vi "Multirecord Acquisition (FPGA)_20220927.vi"() -> ()   [LabVIEW 2021]
doc: "Use this VI as a template for the reconfigurable oscilloscope acquisition design. The block diagram is divided into three main loops.\n\nRegister Bus: This loop initializes the registers that are needed to support the configuration of the device. The FIFO bus, on the left, allows all the other design libraries to communicate with one another. This loop is very important to support the proper behavior of the instrument design library components.\n\nAcquisition: Acquires data from the I/O channels and writes the data into the record memory using the <B>Write</B> VI of the Multirecord Acquisition instrument design library. This VI also evaluates the various acquisition triggers and decides whether to acquire each data value in record memory. The host level VI (Fetch Record.vi) can read acquired records from the DRAM. The data is stored in 2 DRAM banks, each with 768 MB of storage.\n\nFetch: The recorded data is retrieved when the <B>Fetch Single Record</B> VI is run from the host VI. The <B>Write to Fetch DMA FIFO</B> VI writes data to the acq.fetch fifo 0 to transmit record data form the FPGA to the record fetch VIs on the host. This DMA FIFO must have a predefined name based on the instance parameter. By default, it is 0 (since the associated terminal on the <B>Create Resources DRAM Write Read</B> VI is unwired), so the connected FIFO is named acq.fetch fifo 0."
uses:
  <vilib>/Platform/TimedLoop/XDataNode/XDataNode.xnode
  <vilib>/Platform/TimedLoop/XDataNode/nitl_modes.ctl
  <vilib>/Platform/TimedLoop/XDataNode/XDNodeRunTimeDep.lvlib
  <vilib>/Platform/TimedLoop/XDataNode/wakeup.ctl
  <vilib>/Platform/TimedLoop/XDataNode/timing_clust.ctl
  <instrlib>/_niInstr/Multirecord Acquisition/Interface/v1/FPGA/niInstr Multirecord Acquisition v1 FPGA.lvclass
  <instrlib>/_niInstr/Multirecord Acquisition/Common/v1/FPGA/niInstr Multirecord Acquisition Common v1 FPGA.lvclass
  <vilib>/rvi/LocalResourceManager/LocalResourceManager.xnode
  <vilib>/rvi/eio/common/nirviEmuReportErrorAndStop.vi
  <vilib>/rvi/DataTransferAndStorage/Container/Common/niFpgaContainerGetUniqueNameForEmu.vi
  <vilib>/rvi/DataTransferAndStorage/Container/Common/niFpgaContainerSetEmuInfo.vi
  <vilib>/eio/EIONode/EIONode.xnode
  <instrlib>/_niInstr/FIFO Register Bus/v1/FPGA/niInstr FIFO Register Bus v1 FPGA.lvclass
  <instrlib>/_niInstr/Instruction Framework/v1/FPGA/Top Level Bus/Register Configuration/Register Configuration.lvclass
  <instrlib>/_niInstr/Channel/v1/FPGA/niInstr Channel v1 FPGA.lvlib
  <instrlib>/_niInstr/Basic Elements/v1/FPGA/niInstr Basic Elements v1 FPGA.lvlib
  <instrlib>/_niInstr/Multirecord Acquisition/Common/v1/FPGA/Private/Create Fetch DMA FIFO Resources U8x32.vi
  <instrlib>/HSAI-RIO/Config/Group A/v1/FPGA/Digital Correction/Digital Correction.lvclass
  <instrlib>/HSAI-RIO/Config/Group A/v1/FPGA/Config Registers/Config Registers.lvclass
  <instrlib>/_niInstr/Channel/v1/FPGA/Private/Select/Select FXP(+-,18,1,)xNspcx8ch.vi
  Trigger/Trigger FXP(+,-,18,1).vi
  Data Type Conversion/SubVIs/Remove Overflow FXP(+-,18,1)x8ch.vi
  <instrlib>/HSAI-RIO/Config/Group A/v1/FPGA/Digital Correction/FIR Filter (8 Ch).vi
  <instrlib>/_niInstr/Multirecord Acquisition/Interface/v1/FPGA/Private/Retrieve Record U16 Wrapper.vi
  <instrlib>/_niInstr/Multirecord Acquisition/Common/v1/FPGA/Private/Create Resources BRAM U384.vi
  <instrlib>/_niInstr/Multirecord Acquisition/Interface/v1/FPGA/Private/Write to Fetch DMA FIFO U16 Wrapper.vi
  <instrlib>/_niInstr/Multirecord Acquisition/Common/v1/FPGA/Private/Create Resources DRAM U384x2 U768 Write Read.vi
  Emulation/SubVIs/2 Element Generate Sine Cos Data FXP(+,-,14,1).vi
  <instrlib>/HSAI-RIO/Config/Group A/v1/FPGA/Digital Correction/Validate 8 Channel Data.vi
  <instrlib>/HSAI-RIO/Config/Group A/v1/FPGA/Digital Correction/Digital Correction (8 Ch).vi
  <instrlib>/_niInstr/Multirecord Acquisition/Common/v1/FPGA/Private/Create Resources DRAM U384.vi
  Data Type Conversion/SubVIs/Data Type Conversion FXP(+-,18,1) to I16x8ch.vi
  <instrlib>/_niInstr/Multirecord Acquisition/Common/v1/FPGA/Private/Create Resources BRAM U768.vi
  DSP/SubVIs/Integer decimationx8ch.vi
  <instrlib>/_niInstr/Multirecord Acquisition/Interface/v1/FPGA/Private/Write I16 Wrapper.vi
  <instrlib>/_niInstr/Channel/v1/FPGA/Private/Select and Interleave/Select And Interleave I16xNspcx8ch.vi
  C:/Program Files (x86)/National Instruments/LabVIEW 2021/instr.lib/_niInstr/Multirecord Acquisition/Interface/v1/FPGA/niInstr Multirecord Acquisition v1 FPGA.lvclass
  C:/Program Files (x86)/National Instruments/LabVIEW 2021/instr.lib/_niInstr/Multirecord Acquisition/Common/v1/FPGA/niInstr Multirecord Acquisition Common v1 FPGA.lvclass
  <vilib>/rvi/eio/common/nirviEmuTemplateMethod_errors.vi
  C:/Program Files (x86)/National Instruments/LabVIEW 2021/instr.lib/_niInstr/Instruction Framework/v1/FPGA/Interfaces/Instruction Producer/Instruction Producer.lvclass
  C:/Program Files (x86)/National Instruments/LabVIEW 2021/instr.lib/_niInstr/FIFO Register Bus/v1/FPGA/niInstr FIFO Register Bus v1 FPGA.lvclass
  FPGA Interface Typedefinitions/Trigger Combination Type.ctl
  FPGA Interface Typedefinitions/FPGA Interface Typedefinitions.lvlib
  <instrlib>/_niInstr/Data Trigger/v1/Shared/Public/Level Configuration FXP(+-,18,1).ctl
  <instrlib>/_niInstr/Data Trigger/v1/Shared/niInstr Data Trigger v1 Shared.lvlib
  <instrlib>/_niInstr/Data Trigger/v1/Shared/Public/Level Configuration Trigger When.ctl
panel:
  in  "trig 0":cluster{"Hi":T1, "Lo":T1}
  in  "trigger.channel A":u8
  in  "trigger.rearm delay":u16=2
  in  "start trigger":bool=TRUE
  in  "reset":bool
  in  "trigger.combination type":T3
  out "fifo reg bus data 0":u64
  out "fifo reg bus status 0":u32
  in  "fifo reg bus ctrl 0":u32
  out "overflow":bool
  in  "dsp.decimation factor":u16
  out "overload":bool
  in  "channel.enable mask":u16=65535 format="%.0b"
  in  "channel.number of channels":u8=8
  # "Register Bus Controls"
  # "FPGA"
  # "Acquisition Loop Controls"
  # "DSP"
  # "Trigger"
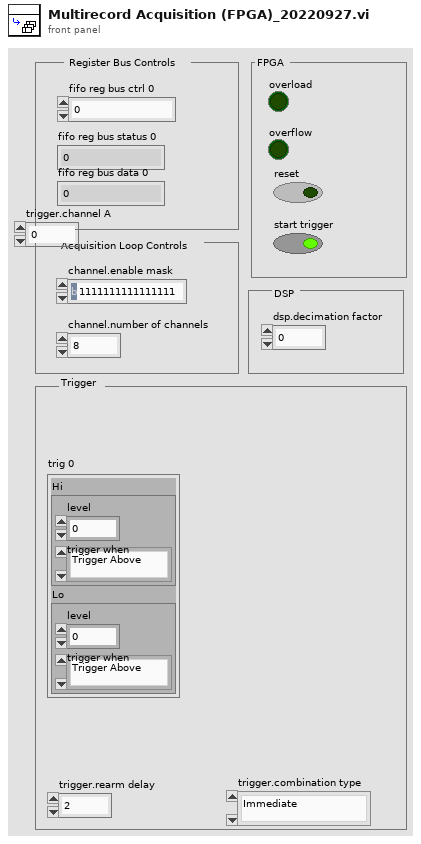
[diagram p1: front panel]
types:
  T1 = typedef "niInstr Data Trigger v1 Shared.lvlib/Level Configuration FXP(+-,18,1).ctl" = cluster{"level":fxp<+/-,18,1>, "trigger when":T2}
  T2 = typedef "niInstr Data Trigger v1 Shared.lvlib/Level Configuration Trigger When.ctl" = enum8{"Trigger Above", "Trigger Below"}
  T3 = typedef "FPGA Interface Typedefinitions.lvlib/Trigger Combination Type.ctl" = enum16{"Immediate", "A", "B", "OR", "AND", "A THEN B", "B THEN A", "High Resolution"}
  T4 = cluster{"memory 1":refnum<k21>, "memory 2":refnum<k21>}
  T5 = typedef "XDNodeRunTimeDep.lvlib/timing_clust.ctl" = cluster{"Expected End [f-1]":u64, "Actual End [f-1]":u64, "Finished Late? [f-1]":bool, "Expected End [i-1]":u64, "Actual End [i-1]":u64, "Finished Late? [i-1]":bool, "Expected Start [i]":u64, "Actual Start [i]":u64, "Expected Start [f]":u64, "Actual Start [f]":u64, "Source Name":string, "Structure Name":string, "Period":i64, "Deadline":i64, "Offset":i64, "Start":i64, "Priority":i32, "Timeout":i32, "Mode":T6, "Wakeup Reason":T7, "Error":errorcluster, "Source Type":string, "Secondary Source Type":string, "Global End Time":u64, "Global Start Time":u64, "Frame Duration":u64, "Iteration Duration":u64, "Assigned CPU":i32, "I/O Scan Engine Mode":u32}
  T6 = typedef "XDNodeRunTimeDep.lvlib/nitl_modes.ctl" = enum32{"No Change", "Process missed periods, maintain original phase", "Discard missed periods, maintain original phase", "Process missed periods, ignore original phase", "Discard missed periods, ignore original phase"}
  T7 = typedef "XDNodeRunTimeDep.lvlib/wakeup.ctl" = enum32{"Normal", "Aborted", "Asynchronous wakeup", "Timing source error", "Timed loop error", "Timeout"}
  T8 = cluster{"sine data":fxp<+/-,14,1>[], "cosine data":fxp<+/-,14,1>[], "sine data":fxp<+/-,14,1>[], "cosine data":fxp<+/-,14,1>[], "sine data":fxp<+/-,14,1>[], "cosine data":fxp<+/-,14,1>[], "sine data":fxp<+/-,14,1>[], "cosine data":fxp<+/-,14,1>[]}
  T9 = cluster{"Channel 0":fxp<+/-,18,1>[], "Channel 1":fxp<+/-,18,1>[], "Channel 2":fxp<+/-,18,1>[], "Channel 3":fxp<+/-,18,1>[], "Channel 4":fxp<+/-,18,1>[], "Channel 5":fxp<+/-,18,1>[], "Channel 6":fxp<+/-,18,1>[], "Channel 7":fxp<+/-,18,1>[]}
  T10 = cluster{"channel 0":fxp<+/-,18,1>[], "channel 1":fxp<+/-,18,1>[], "channel 2":fxp<+/-,18,1>[], "channel 3":fxp<+/-,18,1>[], "channel 4":fxp<+/-,18,1>[], "channel 5":fxp<+/-,18,1>[], "channel 6":fxp<+/-,18,1>[], "channel 7":fxp<+/-,18,1>[]}
  T11 = cluster{"channel 0":i16[], "channel 1":i16[], "channel 2":i16[], "channel 3":i16[], "channel 4":i16[], "channel 5":i16[], "channel 6":i16[], "channel 7":i16[]}
  T12 = typedef "niInstr Multirecord Acquisition v1 FPGA.lvclass/Timestamp.ctl" = cluster{"timestamp":u64, "valid":bool}
  T13 = typedef "niInstr Types v1 Shared.lvlib/Input Triggers.ctl" = cluster{"start":bool, "advance":bool, "reference":bool, "start trigger index":u16, "advance trigger index":u16, "reference trigger index":u16, "reference trigger correction cycle count":u32}
  T14 = typedef "niInstr Types v1 Shared.lvlib/Sample Format.ctl" = cluster{"bits per channel":u16, "samples per clock":u16, "channels":u8}
  T15 = typedef "niInstr Multirecord Acquisition v1 FPGA.lvclass/Events.ctl" = cluster{"ready for start":bool, "ready for advance":bool, "ready for reference":bool, "end of record":bool, "done":bool, "start trigger":bool, "advance trigger":bool, "reference trigger":bool, "start trigger index":u16, "advance trigger index":u16, "reference trigger index":u16}
  T16 = typedef "niInstr Multirecord Acquisition v1 FPGA.lvclass/Retrieve Data Info.ctl" = cluster{"read request size (bits)":u64, "valid data offset (bits)":u16, "valid data size (bits)":u16, "first sample of request":bool, "last sample of request":bool, "Token":T17}
  T17 = typedef "niInstr Types v1 Shared.lvlib/Token.ctl" = cluster{"identifier":u8, "value":u32}
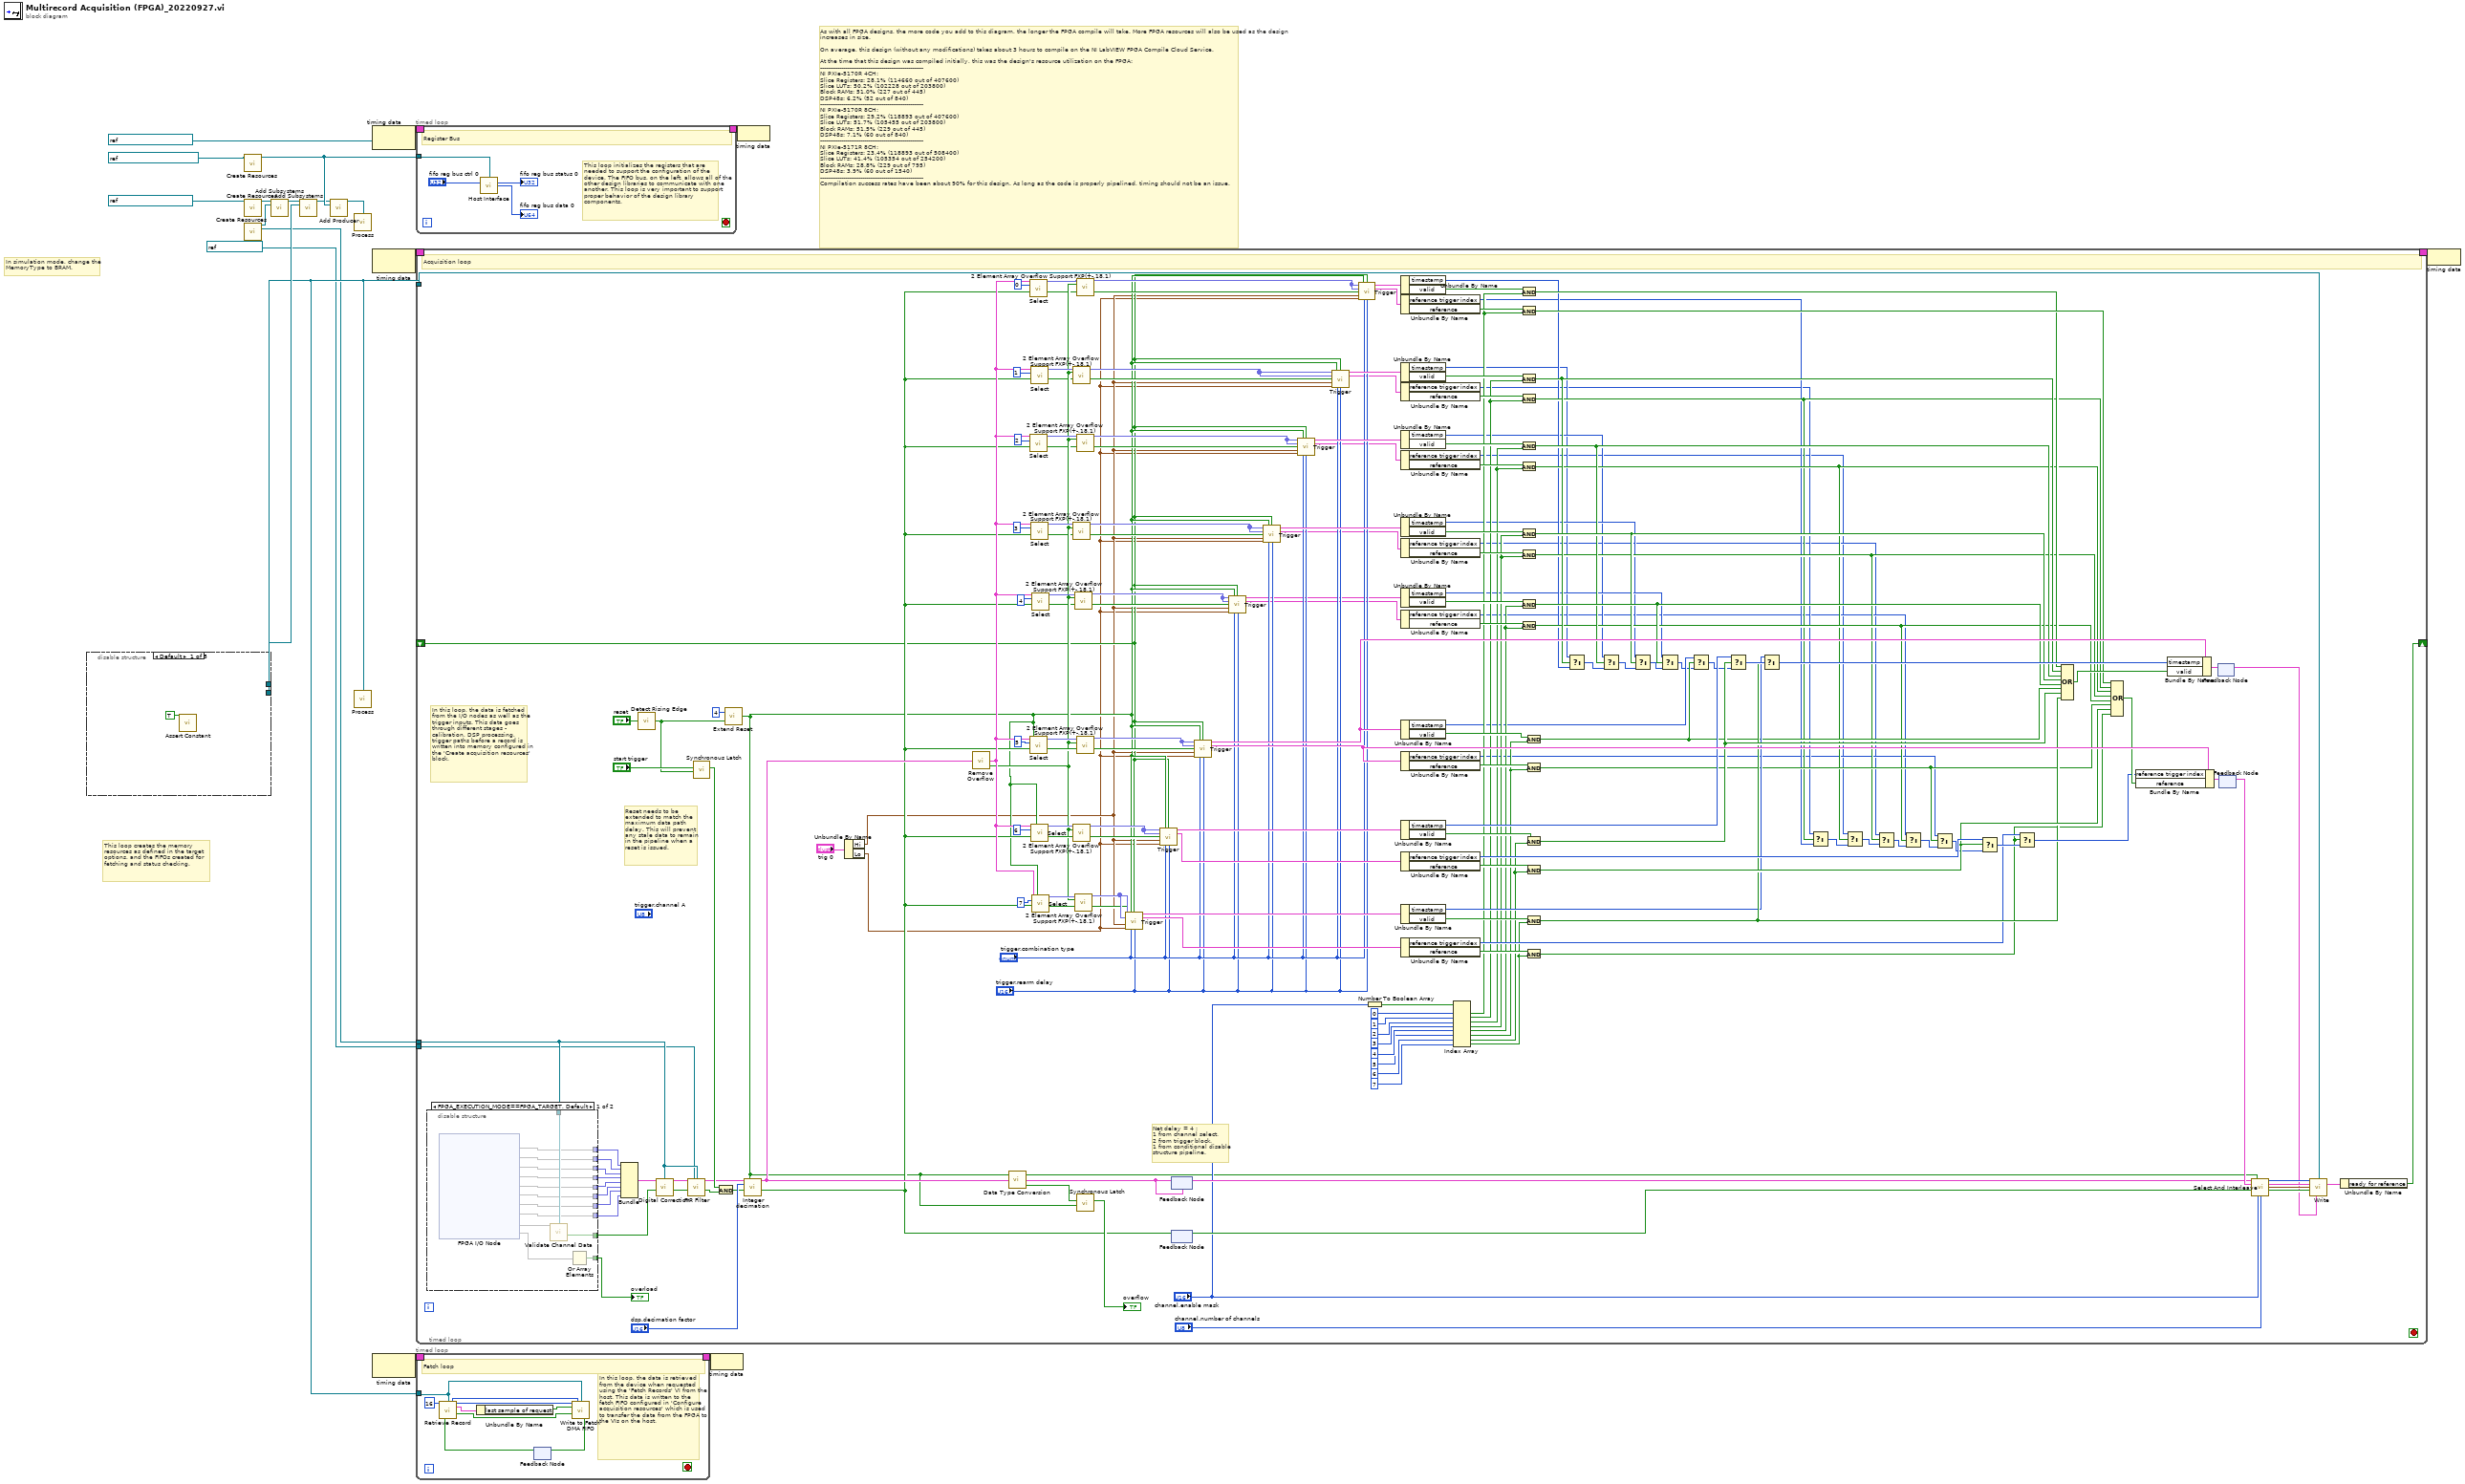
[diagram p0: block diagram]
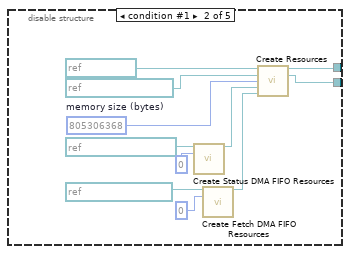
[diagram p2: hidden frame]
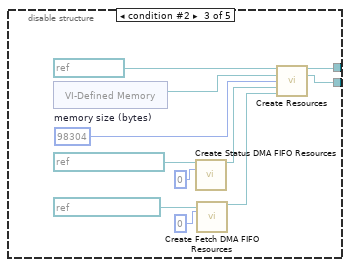
[diagram p3: hidden frame]
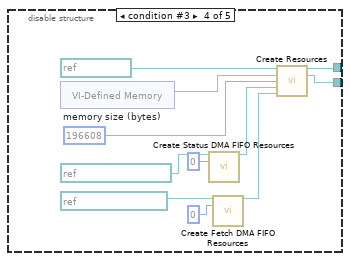
[diagram p4: hidden frame]
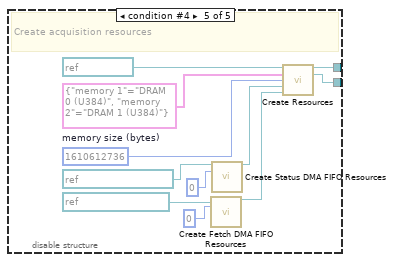
[diagram p5: hidden frame]
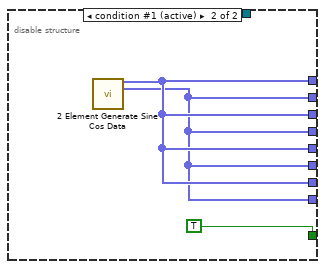
[diagram p6: hidden frame]
diagram:
  # "In simulation mode, change the MemoryType to BRAM."
  # "This loop creates the memory resources as defined in the target options, and the FIFOs created for fetching and status checking."
  # "As with all FPGA designs, the more code you add to this diagram, the longer the FPGA compile will take. More FPGA resources will also be used as the design increases in size.\n\nOn average, this design (without any modifications) takes about 3 hours to compile on the NI LabVIEW FPGA Compile Cloud Service. \n\nAt the time that this design was compiled initially, this was the design's resource utilization on the FPGA:\n------------------------------------------------------\nNI PXIe-5170R 4CH:\nSlice Registers: 28.1% (114660 out of 407600)\nSlice LUTs: 50.2% (102228 out of 203800)\nBlock RAMs: 51.0% (227 out of 445)\nDSP48s: 6.2% (52 out of 840)\n------------------------------------------------------\nNI PXIe-5170R 8CH:\nSlice Registers: 29.2% (118893 out of 407600)\nSlice LUTs: 51.7% (105455 out of 203800)\nBlock RAMs: 51.5% (229 out of 445)\nDSP48s: 7.1% (60 out of 840)\n------------------------------------------------------\nNI PXIe-5171R 8CH:\nSlice Registers: 23.4% (118893 out of 508400)\nSlice LUTs: 41.4% (105354 out of 254200)\nBlock RAMs: 28.8% (229 out of 795)\nDSP48s: 3.9% (60 out of 1540)\n------------------------------------------------------\nCompilation success rates have been about 90% for this design. As long as the code is properly pipelined, timing should not be an issue."
  n1 = disable-structure shown="Default" {
    disable-tunnel: [_ w29 w40 w51 w62] -> w4
    disable-tunnel: [_ w26 w36 w47 w59] -> w7
    frame condition #0 (active) {
      n2 = call <instrlib>:"Assert Constant.vi"("constant terminal"=TRUE) -> ()  [unwired: 15 in]
    }
    frame condition #1 {
      w30 = u64 805306368  # memory size (bytes)
      n3 = call <instrlib>:"Create Status DMA FIFO Resources.vi"("status dma fifo in"=refnum<k21> "acq.status fifo 0" ("status dma fifo"), "fifo instance"=u8 0) -> ("status dma fifo out"=w21:refnum<class "niInstr Status FIFO v1 FPGA.lvclass">)  [unwired: 13 in]
      n4 = call-poly <instrlib>:"Create Fetch DMA FIFO Resources.vi"("fetch dma fifo in"=refnum<k21> "acq.fetch fifo 0", "fifo instance"=u8 0) -> ("fetch dma fifo out"=w27:refnum<class "niInstr Fetch FIFO v1 FPGA.lvclass">)  [unwired: 13 in]
      n5 = call-poly <instrlib>:"Create Resources.vi"("memory clock"=refnum<k21> "160MHz" ("process clock"), "memory"=refnum<k21> "DRAM 0 (U384)" ("dram"), "memory size (bytes)"=w30, "status dma fifo resources"=w21, "fetch dma fifo resources"=w27) -> ("acquisition resources"=w29:refnum<class "niInstr Multirecord Acquisition Common v1 FPGA.lvclass">, "acquisition subsystem"=w26:refnum<class "Address Space Collection.lvclass">)  [unwired: 9 in]
    }
    frame condition #2 {
      w41 = u64 98304  # memory size (bytes)
      n6 = xnode "VI-Defined Memory"() -> ("Memory Out"=w42:refnum<k21>)
      n7 = call <instrlib>:"Create Status DMA FIFO Resources.vi"("status dma fifo in"=refnum<k21> "acq.status fifo 0" ("status dma fifo"), "fifo instance"=u8 0) -> ("status dma fifo out"=w33:refnum<class "niInstr Status FIFO v1 FPGA.lvclass">)  [unwired: 13 in]
      n8 = call-poly <instrlib>:"Create Fetch DMA FIFO Resources.vi"("fetch dma fifo in"=refnum<k21> "acq.fetch fifo 0", "fifo instance"=u8 0) -> ("fetch dma fifo out"=w37:refnum<class "niInstr Fetch FIFO v1 FPGA.lvclass">)  [unwired: 13 in]
      n9 = call-poly <instrlib>:"Create Resources.vi"("memory clock"=refnum<k21> "160MHz" ("process clock"), "memory"=w42, "memory size (bytes)"=w41, "status dma fifo resources"=w33, "fetch dma fifo resources"=w37) -> ("acquisition resources"=w40:refnum<class "niInstr Multirecord Acquisition Common v1 FPGA.lvclass">, "acquisition subsystem"=w36:refnum<class "Address Space Collection.lvclass">)  [unwired: 9 in]
    }
    frame condition #3 {
      w52 = u64 196608  # memory size (bytes)
      n10 = xnode "VI-Defined Memory"() -> ("Memory Out"=w53:refnum<k21>)
      n11 = call <instrlib>:"Create Status DMA FIFO Resources.vi"("status dma fifo in"=refnum<k21> "acq.status fifo 0" ("status dma fifo"), "fifo instance"=u8 0) -> ("status dma fifo out"=w45:refnum<class "niInstr Status FIFO v1 FPGA.lvclass">)  [unwired: 13 in]
      n12 = call-poly <instrlib>:"Create Fetch DMA FIFO Resources.vi"("fetch dma fifo in"=refnum<k21> "acq.fetch fifo 0", "fifo instance"=u8 0) -> ("fetch dma fifo out"=w48:refnum<class "niInstr Fetch FIFO v1 FPGA.lvclass">)  [unwired: 13 in]
      n13 = call-poly <instrlib>:"Create Resources.vi"("memory clock"=refnum<k21> "160MHz" ("process clock"), "memory"=w53, "memory size (bytes)"=w52, "status dma fifo resources"=w45, "fetch dma fifo resources"=w48) -> ("acquisition resources"=w51:refnum<class "niInstr Multirecord Acquisition Common v1 FPGA.lvclass">, "acquisition subsystem"=w47:refnum<class "Address Space Collection.lvclass">)  [unwired: 9 in]
    }
    frame condition #4 {
      w64 = u64 1610612736  # memory size (bytes)
      # "Create acquisition resources"
      n14 = call-poly <instrlib>:"Create Fetch DMA FIFO Resources.vi"("fetch dma fifo in"=refnum<k21> "acq.fetch fifo 0", "fifo instance"=u8 0) -> ("fetch dma fifo out"=w61:refnum<class "niInstr Fetch FIFO v1 FPGA.lvclass">)  [unwired: 13 in]
      n15 = call <instrlib>:"Create Status DMA FIFO Resources.vi"("status dma fifo in"=refnum<k21> "acq.status fifo 0" ("status dma fifo"), "fifo instance"=u8 0) -> ("status dma fifo out"=w56:refnum<class "niInstr Status FIFO v1 FPGA.lvclass">)  [unwired: 13 in]
      n16 = call-poly <instrlib>:"Create Resources.vi"("memory clock"=refnum<k21> "160MHz" ("process clock"), "memory"=T4 {"memory 1"="DRAM 0 (U384)", "memory 2"="DRAM 1 (U384)"}, "memory size (bytes)"=w64, "status dma fifo resources"=w56, "fetch dma fifo resources"=w61) -> ("acquisition resources"=w62:refnum<class "niInstr Multirecord Acquisition Common v1 FPGA.lvclass">, "acquisition subsystem"=w59:refnum<class "Address Space Collection.lvclass">)  [unwired: 9 in]
    }
  }
  n17 = call <instrlib>:"Create Resources.vi"("instruction fifo"=refnum<k21> "reg.host instruction fifo 0" ("FIFO")) -> ("fifo register bus"=w6:refnum<class "niInstr FIFO Register Bus v1 FPGA.lvclass">)  [unwired: 14 in]
  n18 = call <instrlib>:"Create Resources.vi"("register clock"=refnum<k21> "40 MHz Onboard Clock" ("Source Name")) -> ("register configuration"=w10:refnum<class "Register Configuration.lvclass">)  [unwired: 14 in]
  n19 = call <instrlib>:"Create Resources.vi"() -> ("config subsystems"=w8:refnum<class "Address Space Collection.lvclass">, "digital correction resources"=w1:refnum<class "Digital Correction.lvclass">)  [unwired: 14 in]
  n20 = call-dynamic "Add Subsystems.vi"("register configuration in"=w10, "subsystems"=w8) -> ("register configuration out"=w9:refnum<class "Register Configuration.lvclass">)  [unwired: 13 in]
  n21 = call-dynamic "Add Subsystems.vi"("register configuration in"=w9, "subsystems"=w7) -> ("register configuration out"=w3:refnum<class "Register Configuration.lvclass">)  [unwired: 13 in]
  n22 = call-dynamic "Add Producer.vi"("register configuration in"=w3, "instruction producer"=w6) -> ("register configuration out"=w5:refnum<class "Register Configuration.lvclass">)  [unwired: 13 in]
  n23 = call-dynamic "Process.vi"("register configuration"=w5) -> ()  [unwired: 15 in]
  n24 = call-dynamic "Process.vi"("acquisition resources"=w4) -> ()  [unwired: 15 in]
  n25 = node-c288(refnum<k21> "40 MHz Onboard Clock" ("Source Name")) -> (w19:T5)
  n26 = node-c288() -> (w17:T5)  [unwired: 1 in]
  n27 = node-c288() -> (w15:T5)  [unwired: 1 in]
  n28 = timed-loop {
    timing: w19 -> [_]
    timing-out: [_] -> w18
    tunnel: w6 -> [w68]
    stop <- _ stop-if-true
    # "This loop initializes the registers that are needed to support the configuration of the device. The FIFO bus, on the left, allows all of the other design libraries to communicate with one another. This loop is very important to support proper behavior of the design library components."
    # "Register Bus"
    n29 = call <instrlib>:"Host Interface.vi"("fifo register bus"=w68, "fifo reg bus ctrl 0"="fifo reg bus ctrl 0") -> ("fifo reg bus status 0"=→"fifo reg bus status 0":u32, "fifo reg bus data 0"=→"fifo reg bus data 0":u64)  [unwired: 12 in]
  }
  n30 = timed-loop {
    timing: w17 -> [_]
    timing-out: [_] -> w16
    tunnel: w4 -> [w251]
    tunnel: w1 -> [w234]
    shift-right: [w243] -> _
    shift-left: _ -> [w145]
    tunnel: refnum<k21> "Data Clock x2" -> [w231]
    stop <- _ stop-if-true
    # "Net delay = 4 :\n1 from channel select.\n2 from trigger block.\n1 from conditional disable structure pipeline."
    # "Reset needs to be extended to match the maximum data path delay. This will prevent any stale data to remain in the pipeline when a reset is issued."
    # "In this loop, the data is fetched from the I/O nodes as well as the trigger inputs. This data goes through different stages - calibration, DSP processing, trigger paths before a record is written into memory configured in the 'Create acquisition resources' block."
    # "Acquisition loop"
    n31 = disable-structure shown="FPGA_EXECUTION_MODE==FPGA_TARGET, Default" {
      disable-tunnel: [w263 w268] -> w230
      disable-tunnel: [w262 w267] -> w229
      disable-tunnel: [w261 w268] -> w228
      disable-tunnel: [w260 w267] -> w227
      disable-tunnel: [w259 w268] -> w226
      disable-tunnel: [w258 w267] -> w225
      disable-tunnel: [w257 w268] -> w223
      disable-tunnel: [w256 w267] -> w224
      disable-tunnel: [w253 TRUE ("ADC Data Valid")] -> w221
      disable-tunnel: w234 -> [w264 _]
      disable-tunnel: [w254 _] -> w250
      frame condition #0 {
        # "I/O Nodes"
        n32 = xnode "FPGA I/O Node"() -> ("Channel 0"=w263, "Channel 1"=w262, "Channel 2"=w261, "Channel 3"=w260, "Channel 4"=w259, "Channel 5"=w258, "Channel 6"=w257, "Channel 7"=w256, "Channel Data Valid"=w265, "Channel Overload"=w255)  [unwired: 10 in, 10 out]
        n33 = call-poly <instrlib>:"Validate Channel Data.vi"("channel data valid"=w265, "digital correction resources"=w264) -> ("expected data valid"=w253:bool)  [unwired: 13 in]
        n34 = Or Array Elements(Boolean array=w255) -> (logical OR=w254:bool)
      }
      frame condition #1 (active) {
        n35 = call-poly "2 Element Generate Sine Cos Data.vi"() -> ("sine data"=w268:fxp<+/-,14,1>[], "cosine data"=w267:fxp<+/-,14,1>[])  [unwired: 14 in]
      }
    }
    "overload" <- w250
    n36 = Bundle("sine data"=w230, "cosine data"=w229, "sine data"=w228, "cosine data"=w227, "sine data"=w226, "cosine data"=w225, "sine data"=w223, "cosine data"=w224) -> (w222:T8)  [unwired: 1 in]
    n37 = call <instrlib>:"Detect Rising Edge.vi"("signal"="reset") -> ("edge detected"=w233:bool)  [unwired: 14 in]
    n38 = call-poly <instrlib>:"Digital Correction.vi"("channel data in"=w222, "digital correction resources"=w234, "input valid"=w221) -> ("corrected channel data out"=w214:T9, "output valid"=w213:bool)  [unwired: 11 in]
    n39 = call-poly <instrlib>:"FIR Filter.vi"("data in"=w214, "data clock x2"=w231, "digital correction resources"=w234, "input valid"=w213) -> ("data out"=w211:T9, "output valid"=w212:bool)  [unwired: 9 in, 1 out]
    n40 = call <instrlib>:"Synchronous Latch.vi"("clear"=w233, "set"="start trigger") -> ("out"=w239:bool)  [unwired: 9 in]
    n41 = And(x=w239, y=w212) -> (x .and. y?=w215:bool)
    n42 = call "Extend Reset.vi"("reset in"=w233, "number of cycles"=u8 4) -> ("reset out"=w146:bool)
    n43 = call-poly "Integer decimation.vi"("data in"=w211, "reset"=w146, "decimation factor"="dsp.decimation factor", "input valid"=w215) -> ("data out"=w218:T10, "output valid"=w162:bool)  [unwired: 9 in, 1 out]
    n44 = Unbundle By Name("trig 0") -> ("Hi"=w72:T1, "Lo"=w71:T1)
    n45 = call-poly "Remove Overflow.vi"("data in"=w218) -> ("overflow"=w156:bool, "data out"=w168:T10)  [unwired: 3 in]
    n46 = call-poly "Data Type Conversion.vi"("data in"=w218) -> ("overflow"=w220:bool, "data out"=w217:T11)  [unwired: 3 in]
    n47 = call-poly <instrlib>:"Select.vi"("data in"=w168, "channel index"=u8 0 ("trigger.channel A"), "input valid"=w162) -> ("channel out"=w167:fxp<+/-,18,1>[], "output valid"=w151:bool)  [unwired: 11 in]
    n48 = call-poly <instrlib>:"Select.vi"("data in"=w168, "channel index"=u8 2 ("trigger.channel A"), "input valid"=w162) -> ("channel out"=w165:fxp<+/-,18,1>[], "output valid"=w153:bool)  [unwired: 11 in]
    n49 = call-poly <instrlib>:"Select.vi"("data in"=w168, "reset"=w146, "channel index"=u8 5 ("trigger.channel A"), "input valid"=w162) -> ("channel out"=w241:fxp<+/-,18,1>[], "output valid"=w210:bool)  [unwired: 10 in]
    n50 = call-poly <instrlib>:"Select.vi"("data in"=w168, "channel index"=u8 1, "input valid"=w162) -> ("channel out"=w166:fxp<+/-,18,1>[], "output valid"=w152:bool)  [unwired: 11 in]
    n51 = call-poly <instrlib>:"Select.vi"("data in"=w168, "channel index"=u8 3, "input valid"=w162) -> ("channel out"=w164:fxp<+/-,18,1>[], "output valid"=w154:bool)  [unwired: 11 in]
    n52 = call-poly <instrlib>:"Select.vi"("data in"=w168, "reset"=w146, "channel index"=u8 6, "input valid"=w162) -> ("channel out"=w207:fxp<+/-,18,1>[], "output valid"=w205:bool)  [unwired: 10 in]
    n53 = call-poly <instrlib>:"Select.vi"("data in"=w168, "channel index"=u8 4, "input valid"=w162) -> ("channel out"=w163:fxp<+/-,18,1>[], "output valid"=w155:bool)  [unwired: 11 in]
    n54 = call-poly <instrlib>:"Select.vi"("data in"=w168, "reset"=w146, "channel index"=u8 7, "input valid"=w162) -> ("channel out"=w186:fxp<+/-,18,1>[], "output valid"=w184:bool)  [unwired: 10 in]
    n55 = call "2 Element Array Overflow Support FXP(+-,18,1).vi"("data in"=w166, "overflow"=w156) -> ("data out"=w160:fxp<+/-,18,1>[])  [unwired: 13 in]
    n56 = call "2 Element Array Overflow Support FXP(+-,18,1).vi"("data in"=w164, "overflow"=w156) -> ("data out"=w158:fxp<+/-,18,1>[])  [unwired: 13 in]
    n57 = call "2 Element Array Overflow Support FXP(+-,18,1).vi"("data in"=w207, "overflow"=w156) -> ("data out"=w206:fxp<+/-,18,1>[])  [unwired: 13 in]
    n58 = call "2 Element Array Overflow Support FXP(+-,18,1).vi"("data in"=w163, "overflow"=w156) -> ("data out"=w157:fxp<+/-,18,1>[])  [unwired: 13 in]
    n59 = call "2 Element Array Overflow Support FXP(+-,18,1).vi"("data in"=w186, "overflow"=w156) -> ("data out"=w185:fxp<+/-,18,1>[])  [unwired: 13 in]
    n60 = call "2 Element Array Overflow Support FXP(+-,18,1).vi"("data in"=w167, "overflow"=w156) -> ("data out"=w161:fxp<+/-,18,1>[])  [unwired: 13 in]
    n61 = call "2 Element Array Overflow Support FXP(+-,18,1).vi"("data in"=w165, "overflow"=w156) -> ("data out"=w159:fxp<+/-,18,1>[])  [unwired: 13 in]
    n62 = call "2 Element Array Overflow Support FXP(+-,18,1).vi"("data in"=w241, "overflow"=w156) -> ("data out"=w209:fxp<+/-,18,1>[])  [unwired: 13 in]
    n63 = call <instrlib>:"Synchronous Latch.vi"("clear"=w146, "set"=w220) -> ("out"=→"overflow":bool)  [unwired: 9 in]
    n64 = call-poly "Trigger.vi"("data A"=w185, "reset"=w146, "trigger.ready for reference"=w145, "data B"=w185, "input valid"=w184, "trigger.level Hi"=w72, "trigger.level Lo"=w71, "trigger.combination type"="trigger.combination type", "rearm delay"="trigger.rearm delay") -> ("timestamps"=w183:T12, "trigger.out"=w182:T13)  [unwired: 4 in, 1 out]
    n65 = call-poly "Trigger.vi"("data A"=w206, "reset"=w146, "trigger.ready for reference"=w145, "data B"=w206, "input valid"=w205, "trigger.level Hi"=w72, "trigger.level Lo"=w71, "trigger.combination type"="trigger.combination type", "rearm delay"="trigger.rearm delay") -> ("timestamps"=w200:T12, "trigger.out"=w199:T13)  [unwired: 4 in, 1 out]
    n66 = feedback #1(w217) -> (w219:T11)
    n67 = feedback-in #1(w217) -> ()
    n68 = feedback #2() -> (w216:bool)  [unwired: 1 in]
    n69 = feedback-in #2(w162) -> ()
    n70 = call-poly "Trigger.vi"("data A"=w209, "reset"=w146, "trigger.ready for reference"=w145, "data B"=w209, "input valid"=w210, "trigger.level Hi"=w72, "trigger.level Lo"=w71, "trigger.combination type"="trigger.combination type", "rearm delay"="trigger.rearm delay") -> ("timestamps"=w204:T12, "trigger.out"=w202:T13)  [unwired: 4 in, 1 out]
    n71 = call-poly "Trigger.vi"("data A"=w157, "reset"=w146, "trigger.ready for reference"=w145, "data B"=w157, "input valid"=w155, "trigger.level Hi"=w72, "trigger.level Lo"=w71, "trigger.combination type"="trigger.combination type", "rearm delay"="trigger.rearm delay") -> ("timestamps"=w138:T12, "trigger.out"=w137:T13)  [unwired: 4 in, 1 out]
    n72 = call-poly "Trigger.vi"("data A"=w158, "reset"=w146, "trigger.ready for reference"=w145, "data B"=w158, "input valid"=w154, "trigger.level Hi"=w72, "trigger.level Lo"=w71, "trigger.combination type"="trigger.combination type", "rearm delay"="trigger.rearm delay") -> ("timestamps"=w147:T12, "trigger.out"=w139:T13)  [unwired: 4 in, 1 out]
    n73 = call-poly "Trigger.vi"("data A"=w159, "reset"=w146, "trigger.ready for reference"=w145, "data B"=w159, "input valid"=w153, "trigger.level Hi"=w72, "trigger.level Lo"=w71, "trigger.combination type"="trigger.combination type", "rearm delay"="trigger.rearm delay") -> ("timestamps"=w148:T12, "trigger.out"=w140:T13)  [unwired: 4 in, 1 out]
    n74 = call-poly "Trigger.vi"("data A"=w160, "reset"=w146, "trigger.ready for reference"=w145, "data B"=w160, "input valid"=w152, "trigger.level Hi"=w72, "trigger.level Lo"=w71, "trigger.combination type"="trigger.combination type", "rearm delay"="trigger.rearm delay") -> ("timestamps"=w149:T12, "trigger.out"=w141:T13)  [unwired: 4 in, 1 out]
    n75 = call-poly "Trigger.vi"("data A"=w161, "reset"=w146, "trigger.ready for reference"=w145, "data B"=w161, "input valid"=w151, "trigger.level Hi"=w72, "trigger.level Lo"=w71, "trigger.combination type"="trigger.combination type", "rearm delay"="trigger.rearm delay") -> ("timestamps"=w150:T12, "trigger.out"=w142:T13)  [unwired: 4 in, 1 out]
    n76 = Number To Boolean Array(number="channel.enable mask") -> (Boolean array=w195:bool[])
    n77 = Unbundle By Name(w150) -> ("timestamp"=w100:u64, "valid"=w131:bool)
    n78 = Unbundle By Name(w142) -> ("reference trigger index"=w89:u16, "reference"=w130:bool)
    n79 = Unbundle By Name(w149) -> ("timestamp"=w90:u64, "valid"=w129:bool)
    n80 = Unbundle By Name(w141) -> ("reference trigger index"=w88:u16, "reference"=w128:bool)
    n81 = Unbundle By Name(w148) -> ("timestamp"=w91:u64, "valid"=w127:bool)
    n82 = Unbundle By Name(w140) -> ("reference trigger index"=w79:u16, "reference"=w126:bool)
    n83 = Unbundle By Name(w147) -> ("timestamp"=w92:u64, "valid"=w125:bool)
    n84 = Unbundle By Name(w139) -> ("reference trigger index"=w80:u16, "reference"=w124:bool)
    n85 = Unbundle By Name(w138) -> ("timestamp"=w93:u64, "valid"=w123:bool)
    n86 = Unbundle By Name(w137) -> ("reference trigger index"=w81:u16, "reference"=w122:bool)
    n87 = Unbundle By Name(w204) -> ("timestamp"=w99:u64, "valid"=w192:bool)
    n88 = Unbundle By Name(w202) -> ("reference trigger index"=w83:u16, "reference"=w190:bool)
    n89 = Unbundle By Name(w200) -> ("timestamp"=w198:u64, "valid"=w191:bool)
    n90 = Unbundle By Name(w199) -> ("reference trigger index"=w197:u16, "reference"=w189:bool)
    n91 = Unbundle By Name(w183) -> ("timestamp"=w170:u64, "valid"=w180:bool)
    n92 = Unbundle By Name(w182) -> ("reference trigger index"=w169:u16, "reference"=w181:bool)
    n93 = Index Array(array=w195, index #1=0 ("index"), index #2=1 ("index"), index #3=2 ("index"), index #4=3 ("index"), index #5=4 ("index"), index #6=5 ("index"), index #7=6 ("index"), index #8=7 ("index")) -> (element #1=w121:bool, element #2=w120:bool, element #3=w119:bool, element #4=w118:bool, element #5=w117:bool, element #6=w116:bool, element #7=w115:bool, element #8=w114:bool)
    n94 = And(x=w131, y=w121) -> (x .and. y?=w111:bool)
    n95 = And(x=w130, y=w121) -> (x .and. y?=w112:bool)
    n96 = And(x=w129, y=w120) -> (x .and. y?=w106:bool)
    n97 = And(x=w128, y=w120) -> (x .and. y?=w101:bool)
    n98 = And(x=w127, y=w119) -> (x .and. y?=w107:bool)
    n99 = And(x=w126, y=w119) -> (x .and. y?=w102:bool)
    n100 = And(x=w125, y=w118) -> (x .and. y?=w108:bool)
    n101 = And(x=w124, y=w118) -> (x .and. y?=w103:bool)
    n102 = And(x=w123, y=w117) -> (x .and. y?=w109:bool)
    n103 = And(x=w122, y=w117) -> (x .and. y?=w104:bool)
    n104 = And(x=w192, y=w116) -> (x .and. y?=w110:bool)
    n105 = And(x=w190, y=w116) -> (x .and. y?=w105:bool)
    n106 = And(x=w191, y=w115) -> (x .and. y?=w179:bool)
    n107 = And(x=w189, y=w115) -> (x .and. y?=w177:bool)
    n108 = And(x=w180, y=w114) -> (x .and. y?=w171:bool)
    n109 = And(x=w181, y=w114) -> (x .and. y?=w113:bool)
    n110 = Select(t=w90, s=w106, f=w100) -> (s? t:f=w94:u64)
    n111 = Select(t=w91, s=w107, f=w94) -> (s? t:f=w95:u64)
    n112 = Select(t=w92, s=w108, f=w95) -> (s? t:f=w96:u64)
    n113 = Select(t=w93, s=w109, f=w96) -> (s? t:f=w97:u64)
    n114 = Select(t=w99, s=w110, f=w97) -> (s? t:f=w98:u64)
    n115 = Select(t=w198, s=w179, f=w98) -> (s? t:f=w175:u64)
    n116 = Select(t=w170, s=w171, f=w175) -> (s? t:f=w174:u64)
    n117 = Select(t=w88, s=w101, f=w89) -> (s? t:f=w87:u16)
    n118 = Select(t=w79, s=w102, f=w87) -> (s? t:f=w86:u16)
    n119 = Select(t=w80, s=w103, f=w86) -> (s? t:f=w85:u16)
    n120 = Select(t=w81, s=w104, f=w85) -> (s? t:f=w84:u16)
    n121 = Select(t=w83, s=w105, f=w84) -> (s? t:f=w82:u16)
    n122 = Select(t=w197, s=w177, f=w82) -> (s? t:f=w173:u16)
    n123 = Select(t=w169, s=w113, f=w173) -> (s? t:f=w172:u16)
    n124 = Compound Arithmetic op=OR(w111, w106, w107, w108, w109, w110, w179, w171) -> (w178:bool)
    n125 = Compound Arithmetic op=OR(w112, w101, w102, w103, w104, w105, w177, w113) -> (w176:bool)
    n126 = Bundle By Name(cluster=w202, "reference trigger index"=w172, "reference"=w176) -> (w201:T13)
    n127 = Bundle By Name(cluster=w204, "timestamp"=w174, "valid"=w178) -> (w203:T12)
    n128 = feedback #3() -> (w237:T12)  [unwired: 1 in]
    n129 = feedback-in #3(w203) -> ()
    n130 = feedback #4() -> (w238:T13)  [unwired: 1 in]
    n131 = feedback-in #4(w201) -> ()
    n132 = call-poly <instrlib>:"Select And Interleave.vi"("data in"=w219, "reset"=w146, "triggers in"=w238, "input valid"=w216, "channel enable mask"="channel.enable mask", "number of channels to interleave"="channel.number of channels") -> ("interleaved data out"=w249:i16[], "triggers out"=w248:T13, "sample format out"=w247:T14, "output valid"=w246:bool)  [unwired: 5 in, 1 out]
    n133 = call-poly <instrlib>:"Write.vi"("data"=w249, "acquisition resources"=w251, "triggers"=w248, "sample format"=w247, "data valid"=w246, "timestamp"=w237) -> ("events"=w244:T15)  [unwired: 7 in, 2 out]
    n134 = Unbundle By Name(w244) -> ("ready for reference"=w243:bool)
  }
  n135 = timed-loop {
    timing: w15 -> [_]
    timing-out: [_] -> w14
    tunnel: w4 -> [w279]
    stop <- _ stop-if-true
    # "In this loop, the data is retrieved from the device when requested using the 'Fetch Records' VI from the host. This data is written to the fetch FIFO configured in 'Configure acquisition resources' which is used to transfer the data from the FPGA to the VIs on the host."
    # "Fetch loop"
    n136 = feedback #5() -> (w277:bool)  [unwired: 1 in]
    n137 = call-poly <instrlib>:"Retrieve Record.vi"("output array size"=u16 16, "acquisition resources"=w279, "ready for output"=w277) -> ("channels"=w272:u8, "data"=w275:u16[], "retrieve data info"=w274:T16, "output valid"=w276:bool)  [unwired: 9 in]
    n138 = Unbundle By Name(w274) -> ("last sample of request"=w273:bool)
    n139 = call-poly <instrlib>:"Write to Fetch DMA FIFO.vi"("data"=w275, "channels"=w272, "acquisition resources"=w279, "last sample of request"=w273, "input valid"=w276) -> ("ready for input"=w278:bool)  [unwired: 10 in]
    n140 = feedback-in #5(w278) -> ()
  }
  n141 = node-c288(w14) -> ()
  n142 = node-c288(w18) -> ()
  n143 = node-c288(w16) -> ()
